vi "Stop Process.vi"(8 "error in (no error)":errorcluster, 11 "Application in":refnum<class "Application.lvclass">) -> (0 "error out":errorcluster, 3 "Application out":refnum<class "Application.lvclass">)   [LabVIEW 2019, in "Application.lvclass"]
doc: "Developed by Kevin Thompson\nkevin@thompsonengineering.net\n\nCopyright 2018\nThompson Engineering, LLC"
uses:
  Application.lvclass
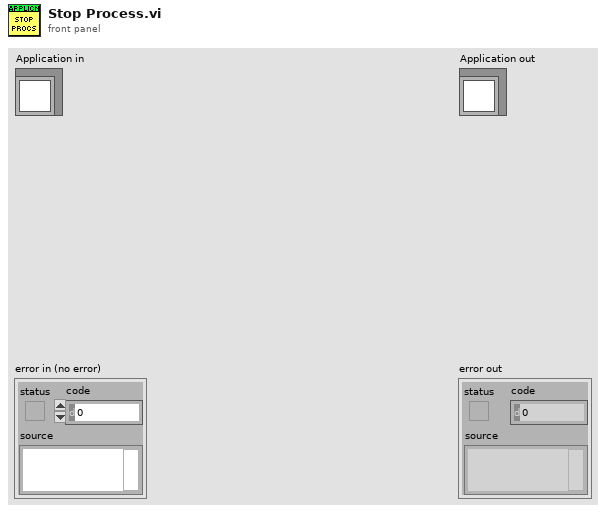
[diagram p1: front panel]
types:
  T1 = typedef "Application.lvclass/Public Events--cluster.ctl" = cluster{"Application.AsyncCmd Event":refnum<user-event>, "Application.AsyncMsg Event":refnum<user-event>, "stop process":refnum<user-event>}
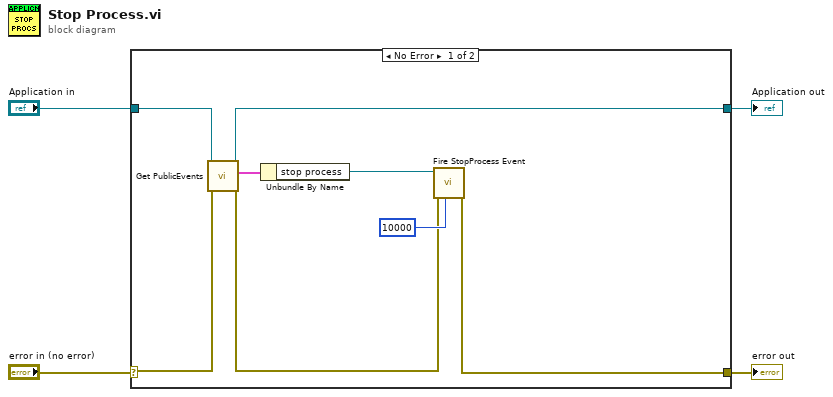
[diagram p0: block diagram]
diagram:
  n1 = case shown="No Error" "error in (no error)" {
    selector: "error in (no error)" -> [w8 w14]
    tunnel: [w12 w14] -> w3
    tunnel: [w10 w13] -> w1
    tunnel: "Application in" -> [w9 w13]
    frame No Error {
      n2 = call "Get PublicEvents.vi"("error in (no error)"=w8, "Application in"=w9) -> ("error out"=w7:errorcluster, "Public Events"=w6:T1, "Application out"=w10:refnum<class "Application.lvclass">)  [unwired: 7 in]
      n3 = Unbundle By Name(w6) -> ("stop process"=w5:refnum<user-event>)
      n4 = call "Fire StopProcess Event.vi"("timeout in ms (5000)"=10000, "error in (no error)"=w7, "Event in"=w5) -> ("error out"=w12:errorcluster)  [unwired: 5 in, 3 out]
    }
    frame Error {
    }
  }
  "error out" <- w3
  "Application out" <- w1
